vi "Create Data Folders.vi"(10 "Experiment Indicator":string, 11 "username":string) -> (3 "Data Output Folder":path)   [LabVIEW 2011]
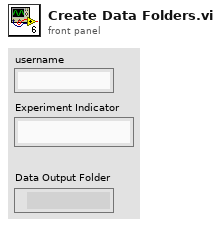
[diagram p1: front panel]
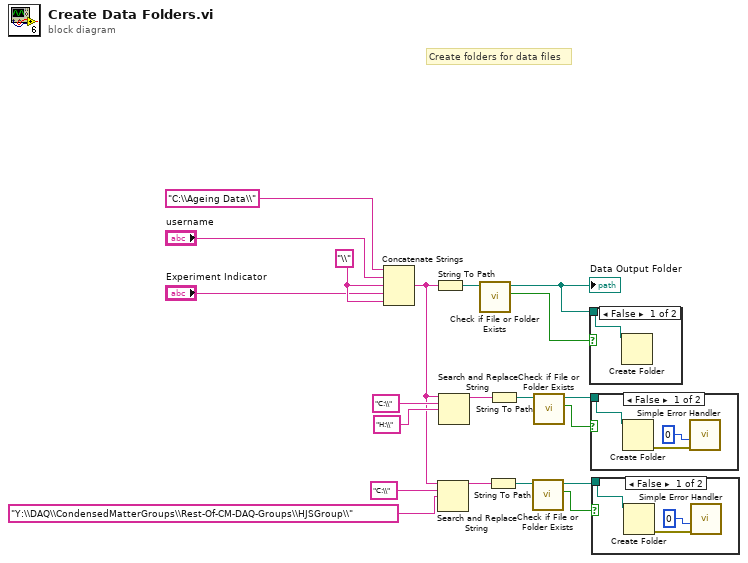
[diagram p0: block diagram]
diagram:
  w10 = "\\"
  # "Create folders for data files"
  n1 = Concatenate Strings("C:\\Ageing Data\\", "username", w10, "Experiment Indicator", w10) -> (w7:string)
  n2 = String To Path(string=w7) -> (path=w19:path)
  n3 = Search and Replace String(input string=w7, search string="C:\\", replace string="Y:\\DAQ\\CondensedMatterGroups\\Rest-Of-CM-DAQ-Groups\\HJSGroup\\") -> (result string=w11:string)  [unwired: 5 in, 3 out]
  n4 = Search and Replace String(input string=w7, search string="C:\\", replace string="H:\\") -> (result string=w15:string)  [unwired: 5 in, 3 out]
  n5 = call <vilib>:"Check if File or Folder Exists.vi"("path"=w19) -> ("file or folder exists?"=w20:bool, "dup path"=w2:path)  [unwired: 8 in, 1 out]
  "Data Output Folder" <- w2
  n6 = String To Path(string=w11) -> (path=w16:path)
  n7 = String To Path(string=w15) -> (path=w17:path)
  n8 = call <vilib>:"Check if File or Folder Exists.vi"("path"=w16) -> ("file or folder exists?"=w3:bool, "dup path"=w4:path)  [unwired: 8 in, 1 out]
  n9 = call <vilib>:"Check if File or Folder Exists.vi"("path"=w17) -> ("file or folder exists?"=w5:bool, "dup path"=w6:path)  [unwired: 8 in, 1 out]
  n10 = case shown="False" w20 {
    tunnel: w2 -> [w21 _]
    frame False {
      n11 = Create Folder(path (use dialog)=w21) -> ()  [unwired: 2 in, 3 out]
    }
    frame True {
    }
  }
  n12 = case shown="False" w5 {
    tunnel: w6 -> [w24 _]
    frame False {
      n13 = Create Folder(path (use dialog)=w24) -> (error out=w23:errorcluster)  [unwired: 2 in, 2 out]
      n14 = call <vilib>:"Simple Error Handler.vi"("type of dialog (OK msg:1)"=0, "error in (no error)"=w23) -> ()  [unwired: 3 in, 5 out]
    }
    frame True {
    }
  }
  n15 = case shown="False" w3 {
    tunnel: w4 -> [w27 _]
    frame False {
      n16 = Create Folder(path (use dialog)=w27) -> (error out=w26:errorcluster)  [unwired: 2 in, 2 out]
      n17 = call <vilib>:"Simple Error Handler.vi"("type of dialog (OK msg:1)"=0, "error in (no error)"=w26) -> ()  [unwired: 3 in, 5 out]
    }
    frame True {
    }
  }
